vi "Configure Harmonics Characteristics.vi"(4 "Select Order (0: All)":i32(ring) items=["All", "Even", "Odd"], 6 "Max Order (0: All)":i32 min=0 max=50, 7 "Item (1)":i32=1 min=1 max=32 step=1, 8 "error in (no error)":errorcluster, 9 "Element (1:1)":i32(ring)=1 items=["1"=1, "2"=2, "3"=3], 10 "Function (0: None)":i32(ring) items=["None", "U", "I", "P", "Phi U", "Phi I", "UHDF", "IHDF", "PHDF"], 11 "VISA resource name":refnum<visa-resource-name>) -> (0 "error out":errorcluster, 3 "VISA resource name out":refnum<visa-resource-name>)   [LabVIEW 2016, in "Yokogawa WT300 Series.lvlib"]
doc: "Configures the Harmonics numeric features."
uses:
  Yokogawa WT300 Series.lvlib
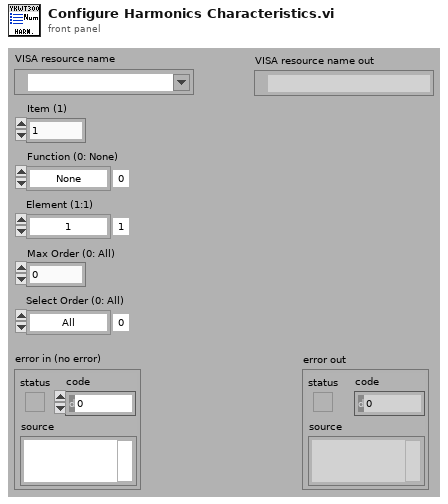
[diagram p1: front panel]
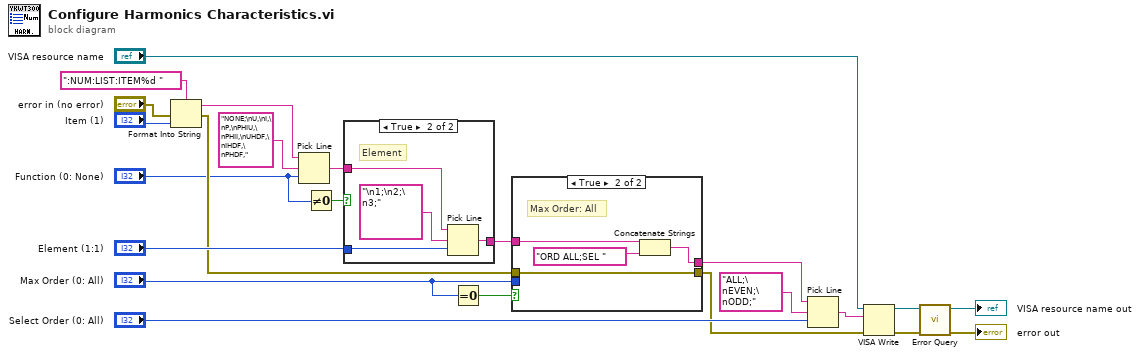
[diagram p0: block diagram]
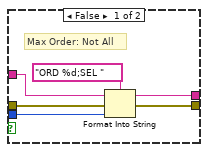
[diagram p3: hidden frame]
diagram:
  n1 = Format Into String(format string=":NUM:LIST:ITEM%d " ("Œ`Ž®•¶Žš—ñ"), error in="error in (no error)", "Item (1)") -> (resulting string=w14:string, error out=w8:errorcluster)  [unwired: 1 in]
  n2 = Pick Line ("ライン選択")(string ("")=w14, multi-line string="NONE;\nU,\nI,\nP,\nPHIU,\nPHII,\nUHDF,\nIHDF,\nPHDF," ("¡s¶ñ"), line index="Function (0: None)") -> (output string=w13:string)
  n3 = Not Equal To 0?(x="Function (0: None)") -> (x != 0?=w2:bool)
  n4 = case shown="True" w2 {
    tunnel: w13 -> [w24 w27]
    tunnel: "Element (1:1)" -> [_ w26]
    tunnel: [w24 w25] -> w9
    frame False {
      # "Function: None"
    }
    frame True {
      # "Element"
      n5 = Pick Line ("ライン選択")(string ("")=w27, multi-line string="\n1;\n2;\n3;" ("¡s¶ñ"), line index=w26) -> (output string=w25:string)
    }
  }
  n6 = Equal To 0?(x="Max Order (0: All)") -> (x = 0?=w11:bool)
  n7 = case shown="True" w11 {
    tunnel: "Max Order (0: All)" -> [w33 _]
    tunnel: w9 -> [w32 w37]
    tunnel: w8 -> [w31 w35]
    tunnel: [w30 w36] -> w6
    tunnel: [w29 w35] -> w3
    frame False {
      # "Max Order: Not All"
      n8 = Format Into String(format string="ORD %d;SEL " ("Œ`Ž®•¶Žš—ñ"), initial string=w32, error in=w31, w33) -> (resulting string=w30:string, error out=w29:errorcluster)
    }
    frame True {
      # "Max Order: All"
      n9 = Concatenate Strings(w37, "ORD ALL;SEL " ("•¶Žš—ñ")) -> (w36:string)
    }
  }
  n10 = Pick Line ("ライン選択")(string ("")=w6, multi-line string="ALL;\nEVEN;\nODD;" ("¡s¶ñ"), line index="Select Order (0: All)") -> (output string=w4:string)
  n11 = VISA Write ("VISA書き込み")(VISA resource name="VISA resource name", write buffer=w4, error in (no error)=w3) -> (VISA resource name out=w23:refnum<visa-resource-name>, error out=w22:errorcluster)  [unwired: 1 out]
  n12 = call "Error Query.vi"("error in (no error)"=w22, "VISA resource name"=w23) -> ("error out"=→"error out":errorcluster, "VISA resource name out"=→"VISA resource name out":refnum<visa-resource-name>)  [unwired: 6 in, 2 out]
